vi "Get Sequence Info.vi"(8 "error in (no error)":errorcluster, 11 "Sequence File Path in":path) -> (0 "error out":errorcluster, 1 "Return Variable":T2, 2 "Parameters":T5[](array[typedef]), 3 "Sequence File Path out":path, 4 "Version":T1, 5 "Description":string)   [LabVIEW 2020, in "NI_VS Sequence Execution Interface.lvlib"]
doc: "Returns information about a sequence in a stimulus profile session."
uses:
  <vilib>/NI VeriStand/Execution/SequenceExecutionInterface/NI_VS Sequence Execution Interface.lvlib
  <vilib>/NI VeriStand/Execution/SequenceExecutionInterface/Input Info.ctl
  <vilib>/NI VeriStand/Execution/SequenceExecutionInterface/Variable Info.ctl
  <vilib>/NI VeriStand/Execution/SequenceExecutionInterface/Type Descriptor Element.ctl
  <vilib>/NI VeriStand/Execution/SequenceExecutionInterface/Data Type.ctl
  <vilib>/NI VeriStand/Execution/SequenceExecutionInterface/Version Info.ctl
  NationalInstruments.VeriStand.RealTimeSequenceDefinitionApi
  NationalInstruments.VeriStand.DataTypes
  NationalInstruments.VeriStand
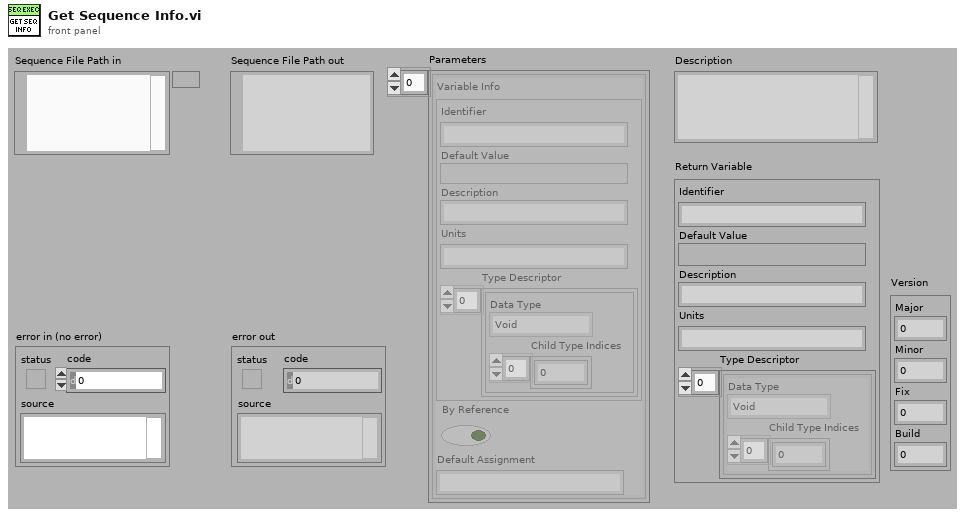
[diagram p1: front panel]
types:
  T1 = typedef "NI_VS Sequence Execution Interface.lvlib/Version Info.ctl" = cluster{"Major":u32, "Minor":u32, "Fix":u32, "Build":u32}
  T2 = typedef "NI_VS Sequence Execution Interface.lvlib/Variable Info.ctl" = cluster{"Identifier":string, "Default Value":variant, "Description":string, "Units":string, "Type Descriptor":T3[]}
  T3 = typedef "NI_VS Sequence Execution Interface.lvlib/Type Descriptor Element.ctl" = cluster{"Data Type":T4, "Child Type Indices":i32[]}
  T4 = typedef "NI_VS Sequence Execution Interface.lvlib/Data Type.ctl" = enum16{"Void", "Boolean", "Int32", "UInt32", "Int64", "UInt64", "Double", "Array"}
  T5 = typedef "NI_VS Sequence Execution Interface.lvlib/Input Info.ctl" = cluster{"Variable Info":T2, "By Reference":bool, "Default Assignment":string}
  T6 = typedef "NI_VS Sequence Execution Interface.lvlib/Data Value Ref.ctl" = refnum<k24>
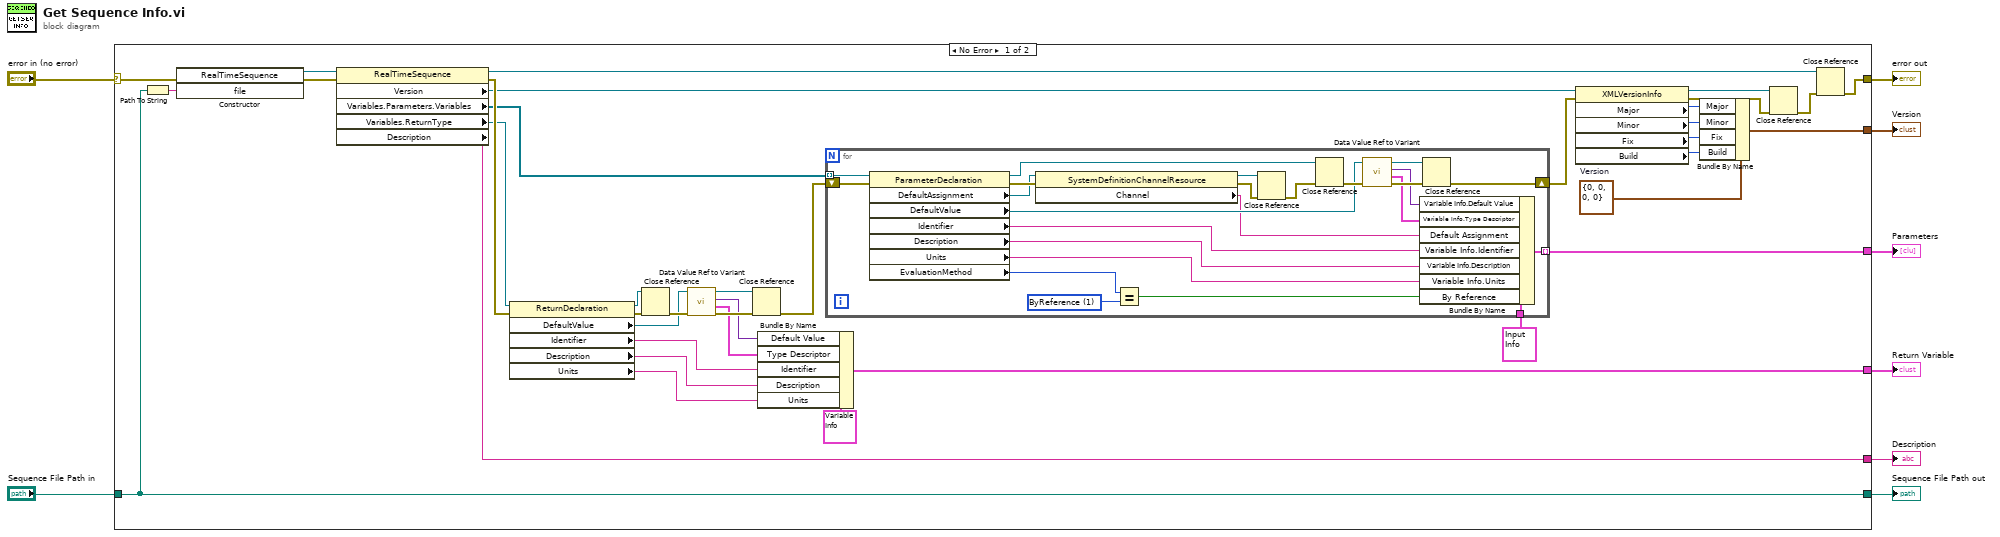
[diagram p0: block diagram]
diagram:
  n1 = case shown="No Error" "error in (no error)" {
    selector: "error in (no error)" -> [w43 w71]
    tunnel: "Sequence File Path in" -> [w41 w72]
    tunnel: [w41 w72] -> w6
    tunnel: [w9 _] -> w5
    tunnel: [w28 w71] -> w4
    tunnel: [w32 _] -> w3
    tunnel: [w31 _] -> w2
    tunnel: [w22 _] -> w1
    frame No Error {
      w19 = T1 {"Major"=0, "Minor"=0, "Fix"=0, "Build"=0}  # Version
      n2 = Path To String(path=w41) -> (string=w42:string)
      n3 = constructor class="RealTimeSequence"(error in=w43, "file"=w42) -> (reference out=w16:refnum<k24>, error out=w15:errorcluster)  [unwired: 2 in, 2 out]
      n4 = property class="RealTimeSequence"(reference=w16, error in=w15) -> (reference out=w14:refnum<k24>, error out=w13:errorcluster, "Version"=w11:refnum<k24>, "Variables.Parameters.Variables"=w12:refnum<k24>[], "Variables.ReturnType"=w10:refnum<k24>, "Description"=w9:string)
      n5 = property class="ReturnDeclaration"(reference=w10, error in=w13) -> (reference out=w37:refnum<k24>, error out=w38:errorcluster, "DefaultValue"=w39:refnum<k24>, "Identifier"=w35:string, "Description"=w34:string, "Units"=w33:string)
      n6 = Close Reference(reference=w37, error in (no error)=w38) -> (error out=w44:errorcluster)
      n7 = call <vilib>:"Data Value Ref to Variant.vi"("error in (no error)"=w44, "Data Value Ref"=w39) -> ("error out"=w45:errorcluster, "Type Descriptor"=w17:T3[], "Variant"=w36:variant, "Data Value Ref out"=w30:T6)  [unwired: 6 in]
      n8 = Close Reference(reference=w30, error in (no error)=w45) -> (error out=w29:errorcluster)
      n9 = Bundle By Name(cluster=T2 {"Identifier"="", "Default Value"=variant, "Description"="", "Units"="", "Type Descriptor"=[]} ("Return Variable"), "Default Value"=w36, "Type Descriptor"=w17, "Identifier"=w35, "Description"=w34, "Units"=w33) -> (w32:T2)
      n10 = for {
        tunnel: w12 -> [w60] mode=indexing
        tunnel: [w59] -> w31 mode=indexing
        shift-right: [w56] -> w20
        shift-left: w29 -> [w58]
        tunnel: T5 {"Variable Info"={"Identifier"="", "Default Value"=variant, "Description"="", "Units"="", "Type Descriptor"=[]}, "By Reference"=FALSE, "Default Assignment"=""} ("Input Info") -> [w55]
        w48 = 1 items=["ByValue", "ByReference"] ("EvaluationMethod")
        n11 = property class="ParameterDeclaration"(reference=w60, error in=w58) -> (reference out=w62:refnum<k24>, error out=w70:errorcluster, "DefaultAssignment"=w53:refnum<k24>, "DefaultValue"=w61:refnum<k24>, "Identifier"=w65:string, "Description"=w66:string, "Units"=w67:string, "EvaluationMethod"=w49:i32)
        n12 = property class="SystemDefinitionChannelResource"(reference=w53, error in=w70) -> (reference out=w54:refnum<k24>, error out=w51:errorcluster, "Channel"=w52:string)
        n13 = Equal?(x=w49, y=w48) -> (x = y?=w47:bool)
        n14 = Close Reference(reference=w54, error in (no error)=w51) -> (error out=w50:errorcluster)
        n15 = Close Reference(reference=w62, error in (no error)=w50) -> (error out=w68:errorcluster)
        n16 = call <vilib>:"Data Value Ref to Variant.vi"("error in (no error)"=w68, "Data Value Ref"=w61) -> ("error out"=w69:errorcluster, "Type Descriptor"=w64:T3[], "Variant"=w63:variant, "Data Value Ref out"=w57:T6)  [unwired: 6 in]
        n17 = Bundle By Name(cluster=w55, "Variable Info.Default Value"=w63, "Variable Info.Type Descriptor"=w64, "Default Assignment"=w52, "Variable Info.Identifier"=w65, "Variable Info.Description"=w66, "Variable Info.Units"=w67, "By Reference"=w47) -> (w59:T5)
        n18 = Close Reference(reference=w57, error in (no error)=w69) -> (error out=w56:errorcluster)
      }
      n19 = property class="XMLVersionInfo"(reference=w11, error in=w20) -> (reference out=w21:refnum<k24>, error out=w46:errorcluster, "Major"=w26:u32, "Minor"=w25:u32, "Fix"=w24:u32, "Build"=w23:u32)
      n20 = Bundle By Name(cluster=w19, "Major"=w26, "Minor"=w25, "Fix"=w24, "Build"=w23) -> (w22:T1)
      n21 = Close Reference(reference=w21, error in (no error)=w46) -> (error out=w18:errorcluster)
      n22 = Close Reference(reference=w14, error in (no error)=w18) -> (error out=w28:errorcluster)
    }
    frame Error {
    }
  }
  "error out" <- w4
  "Parameters" <- w2
  "Sequence File Path out" <- w6
  "Return Variable" <- w3
  "Description" <- w5
  "Version" <- w1
